vi "End.vi"(8 "error in (no error)":errorcluster, 11 "SPARC4_GUI in":refnum<class "S4GEI.lvclass">) -> (0 "error out":errorcluster, 3 "SPARC4_GUI out":refnum<class "S4GEI.lvclass">)   [LabVIEW 2018, in "S4GEI.lvclass"]
uses:
  S4GEI.lvclass
  S4GEI.lvclass/S4GEI.ctl
  Channel GUI/Channel.lvclass
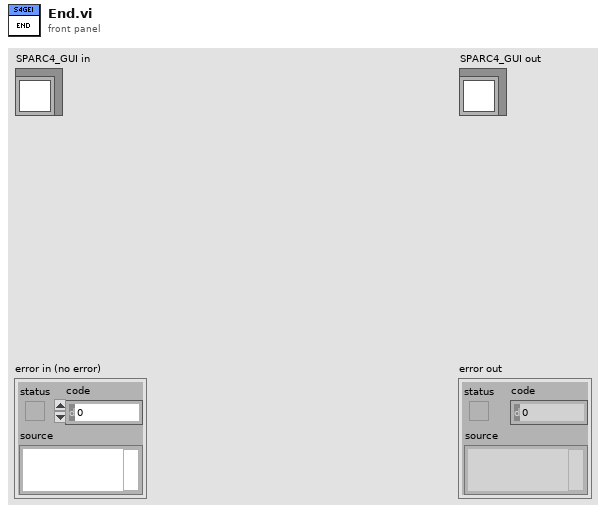
[diagram p1: front panel]
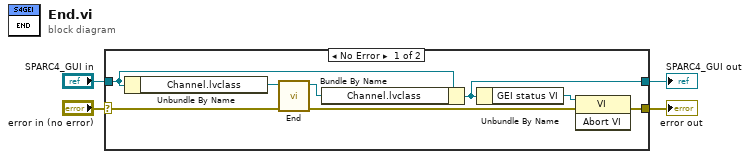
[diagram p0: block diagram]
diagram:
  n1 = case shown="No Error" "error in (no error)" {
    selector: "error in (no error)" -> [w9 w14]
    tunnel: [w6 w14] -> w3
    tunnel: [w5 w13] -> w1
    tunnel: "SPARC4_GUI in" -> [w12 w13]
    frame No Error {
      n2 = Unbundle By Name(w12) -> ("Channel.lvclass"=w11:refnum<class "Channel.lvclass">)
      n3 = call "End.vi"("error in (no error)"=w9, "Channel GUI in"=w11) -> ("error out"=w7:errorcluster, "Channel GUI out"=w10:refnum<class "Channel.lvclass">)  [unwired: 8 in]
      n4 = Bundle By Name(cluster=w12, "Channel.lvclass"=w10) -> (w5:refnum<class "S4GEI.lvclass">)
      n5 = Unbundle By Name(w5) -> ("GEI status VI"=w8:refnum<vi>)
      n6 = invoke class="VI" method="Abort VI"(reference=w8, error in=w7) -> (error out=w6:errorcluster)  [unwired: 1 in, 2 out]
    }
    frame Error {
    }
  }
  "error out" <- w3
  "SPARC4_GUI out" <- w1
